vi "Demarcate.vi"(7 "Mode":enum16{"Read", "Write"}(ring)=enum."Write", 8 "error in":errorcluster, 11 "Sensor IN":T1) -> (0 "error out":errorcluster, 3 "Sensor OUT":T1)   [LabVIEW 2020]
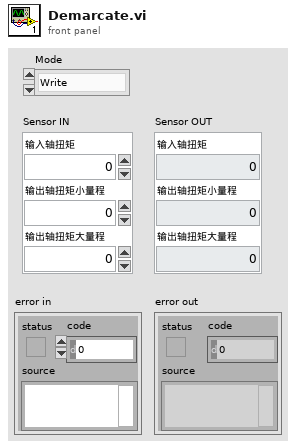
[diagram p1: front panel]
types:
  T1 = cluster{"输入轴扭矩":dbl, "输出轴扭矩小量程":dbl, "输出轴扭矩大量程":dbl}
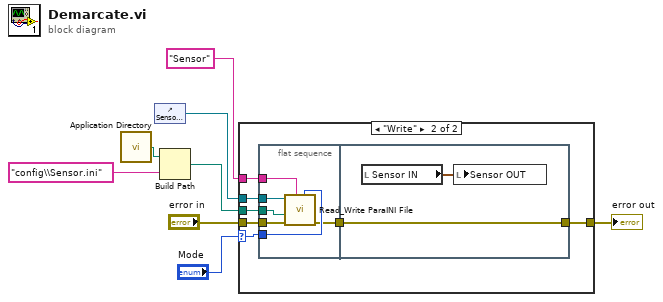
[diagram p0: block diagram]
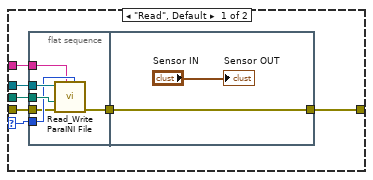
[diagram p2: hidden frame]
diagram:
  n1 = call <vilib>:"Application Directory.vi"() -> ("Application Directory"=w6:path)
  n2 = control-ref of="Sensor IN"() -> (w7:refnum<vi>)
  n3 = Build Path(base path=w6, name or relative path="config\\Sensor.ini" ("名称或相对路径")) -> (appended path=w4:path)
  n4 = case shown="\"Write\"" "Mode" {
    selector: "Mode" -> [w13 w27]
    tunnel: w7 -> [w14 w30]
    tunnel: "Sensor" ("Section") -> [w12 w29]
    tunnel: w4 -> [w15 w28]
    tunnel: "error in" -> [w11 w26]
    tunnel: [w10 w25] -> w1
    frame "Read", Default {
      n5 = flat-sequence {
        tunnel: w15 -> [w21]
        tunnel: w14 -> [w20]
        tunnel: w13 -> [w19]
        tunnel: w12 -> [w18]
        tunnel: w11 -> [w17]
        tunnel: [w16] -> w9
        tunnel: [w23] -> w10
        tunnel: w9 -> [w23]
        frame #0 {
          n6 = call "Read_Write ParaINI File.vi"("Mode"=w19, "Section"=w18, "error in"=w17, "Filepath"=w21, "Ctl Refnum"=w20) -> ("error out"=w16:errorcluster)  [unwired: 6 in]
        }
        frame #1 {
          "Sensor OUT" <- "Sensor IN"
        }
      }
    }
    frame "Write" {
      n7 = flat-sequence {
        tunnel: w30 -> [w36]
        tunnel: w29 -> [w35]
        tunnel: w28 -> [w34]
        tunnel: w27 -> [w33]
        tunnel: w26 -> [w32]
        tunnel: [w31] -> w24
        tunnel: [w38] -> w25
        tunnel: w24 -> [w38]
        frame #0 {
          n8 = call "Read_Write ParaINI File.vi"("Mode"=w33, "Section"=w35, "error in"=w32, "Filepath"=w34, "Ctl Refnum"=w36) -> ("error out"=w31:errorcluster)  [unwired: 6 in]
        }
        frame #1 {
          n9 = local read "Sensor IN"() -> (w37:T1)
          n10 = local write "Sensor OUT"(w37) -> ()
        }
      }
    }
  }
  "error out" <- w1
